vi "Is Feature Toggle Set.vi"(8 "error in (no error)":errorcluster, 11 "Feature Toggle":string) -> (0 "error out":errorcluster, 3 "Is Set":bool)   [LabVIEW 2019, in "grpc-lvsupport.lvlib"]
uses:
  grpc-lvsupport.lvlib
  <resource>/libgrpc_labview.dll
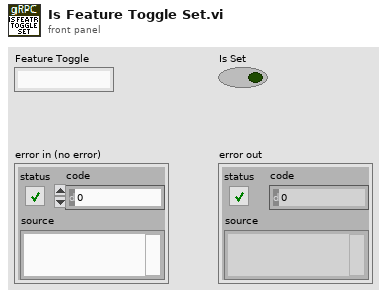
[diagram p1: front panel]
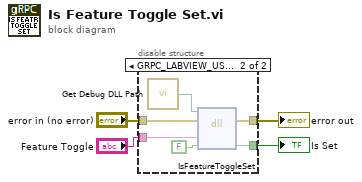
[diagram p0: block diagram]
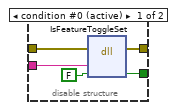
[diagram p2: hidden frame]
diagram:
  n1 = disable-structure shown="GRPC_LABVIEW_USE_DEBUG_DLL==True&&RUN_TIME_ENGINE==False" {
    disable-tunnel: [w9 w15] -> w4
    disable-tunnel: [w8 w14] -> w3
    disable-tunnel: "error in (no error)" -> [w6 w12]
    disable-tunnel: "Feature Toggle" -> [w5 w11]
    frame condition #0 (active) {
      n2 = dll-call lib="C:/Program Files (x86)/National Instruments/LabVIEW 2024/resource/libgrpc_labview.*" fn="IsFeatureToggleSet"(error in=w6, "Feature"=w5, "isSet"=FALSE) -> (error out=w8:errorcluster, "isSet"=w9:bool)  [unwired: 4 in, 1 out]
    }
    frame condition #1 {
      n3 = call "Get Debug DLL Path.vi"() -> ("DLL Path"=w10:path)
      n4 = dll-call lib="?" fn="IsFeatureToggleSet"(path in=w10, error in=w12, "Feature"=w11, "isSet"=FALSE) -> (error out=w14:errorcluster, "isSet"=w15:bool)  [unwired: 3 in, 1 out]
    }
  }
  "Is Set" <- w4
  "error out" <- w3
